vi "Read slope length.vi"(8 "error in (no error)":errorcluster caption="에러 입력(에러 없음)", 11 "Square Wave 입력":refnum<class "Square Wave.lvclass">) -> (0 "error out":errorcluster caption="에러 출력", 2 "slope length":u32, 3 "Square Wave 출력":refnum<class "Square Wave.lvclass">)   [LabVIEW 2020, in "Square Wave.lvclass"]
uses:
  Square Wave.lvclass
  Square Wave.lvclass/Square Wave.ctl
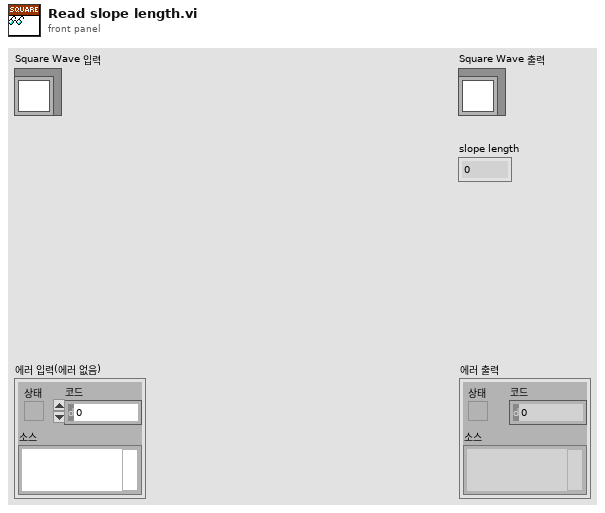
[diagram p1: front panel]
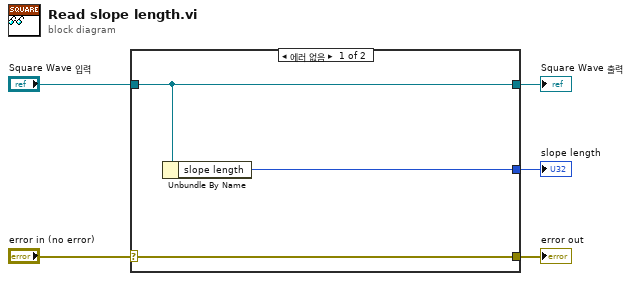
[diagram p0: block diagram]
diagram:
  n1 = case shown="에러 없음" "error in (no error)" {
    selector: "error in (no error)" -> [w8 w9]
    tunnel: [w8 w9] -> w4
    tunnel: [w7 w10] -> w2
    tunnel: "Square Wave 입력" -> [w7 w10]
    tunnel: [w6 _] -> w1
    frame No Error {
      n2 = Unbundle By Name(w7) -> ("slope length"=w6:u32)
    }
    frame Error {
    }
  }
  "error out" <- w4
  "Square Wave 출력" <- w2
  "slope length" <- w1
